vi "Main.vi"() -> ()   [LabVIEW 2024, in "Application.lvlib"]
doc: "This VI is the main application VI in the DQMH project template. This application VI is implemented as a simple state machine, which communicates with two different DQMH modules.\n_____\nBased on DQMH Dev Tools: Project Template 7.1.0.1503."
uses:
  Application.lvlib
  Application Data--cluster.ctl
  State--enum.ctl
  <vilib>/Utility/error.llb/DialogType.ctl
  Camera/Camera.lvlib
  GUI/GUI.lvlib
panel:
  in  "About DQMH":bool
  out "version":string
  in  "Hide GUI Module":bool
  in  "Show GUI Module":bool
  in  "Hide Camera Module":bool
  in  "Show Camera Module":bool
  in  "Stop Camera Module":bool
  in  "Stop GUI Module":bool
  in  "Start GUI Module":bool
  out "Active Camera Modules":string[](array[string])
  in  "Start New Instance Camera Module":bool
  in  "Select Camera Module Instance":i32(ring)=-1 items=["All"=-1, "1"=1]
  out "GUI Running?":bool
  out "Status":string
  # "This top-level application allows you to launch and control a singleton module, and multiple instances of a cloneable module."
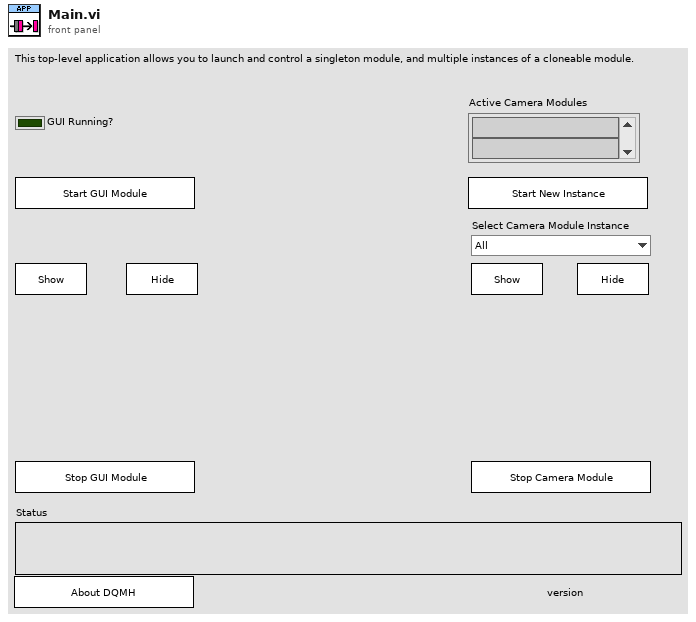
[diagram p1: front panel]
types:
  T1 = typedef "Application.lvlib/State--enum.ctl" = enum16{"Initialize", "Initialize Panel", "UI Interlocks", "Update Status", "Wait for Event", "Exit"}
  T2 = typedef "Application.lvlib/Application Data--cluster.ctl" = cluster{"Status":string, "Singleton Controls":refnum<vi>[], "Cloneable Controls":refnum<vi>[], "Module Ring Value":i32}
  T3 = typedef "Camera.lvlib/Broadcast Events--cluster.ctl" = cluster{"Module Did Init":refnum<user-event>, "Status Updated":refnum<user-event>, "Error Reported":refnum<user-event>, "Module Did Stop":refnum<user-event>, "Update Module Execution Status":refnum<user-event>}
  T4 = typedef "GUI.lvlib/Broadcast Events--cluster.ctl" = cluster{"Module Did Init":refnum<user-event>, "Status Updated":refnum<user-event>, "Error Reported":refnum<user-event>, "Module Did Stop":refnum<user-event>, "Update Module Execution Status":refnum<user-event>, "Update References":refnum<user-event>}
  T5 = enum8{"Enabled", "Disabled", "Disabled and Grayed Out"}
  T6 = typedef "DialogType.ctl" = u16
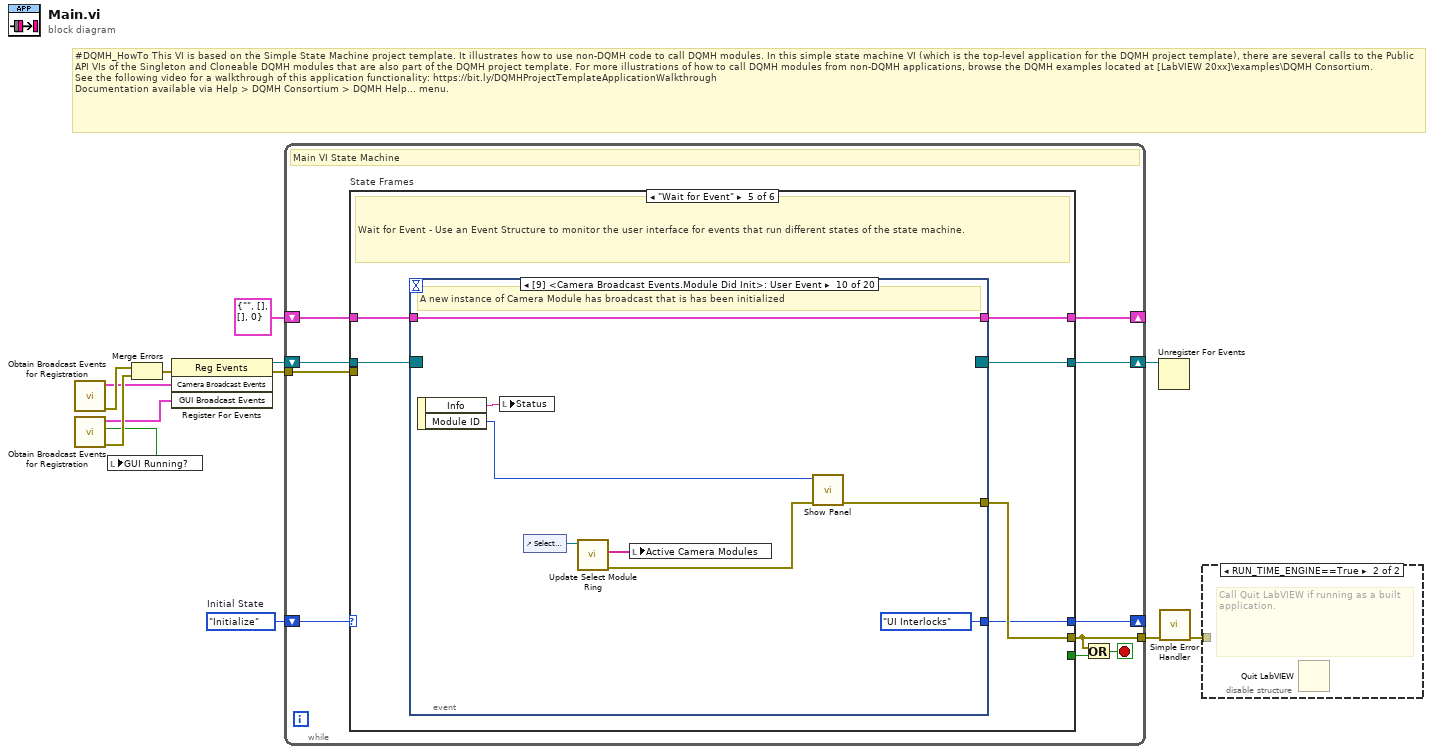
[diagram p0: block diagram]
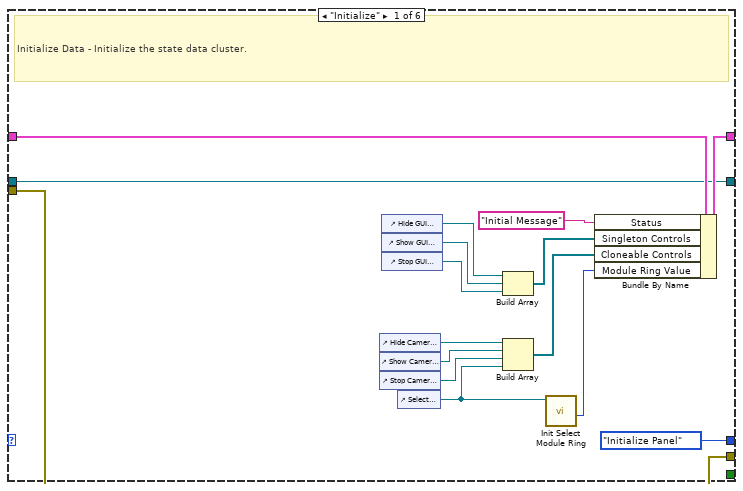
[diagram p2: hidden frame]
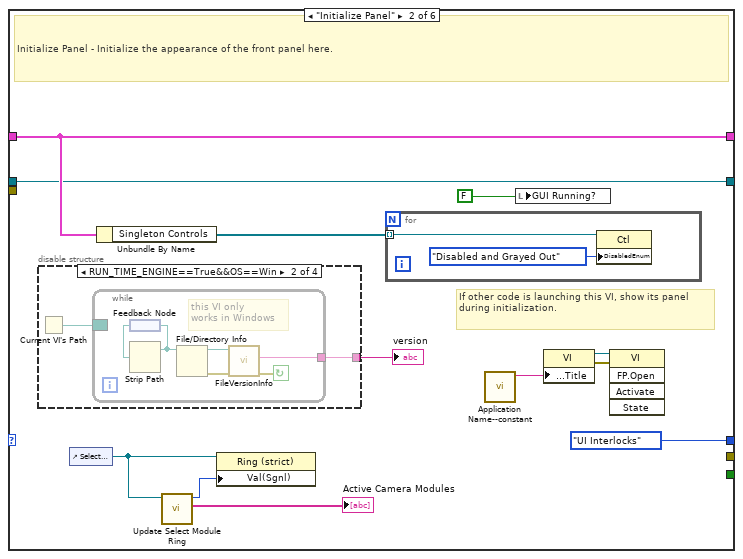
[diagram p3: hidden frame]
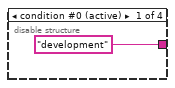
[diagram p4: hidden frame]
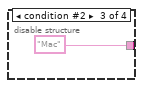
[diagram p5: hidden frame]
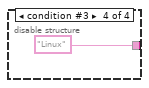
[diagram p6: hidden frame]
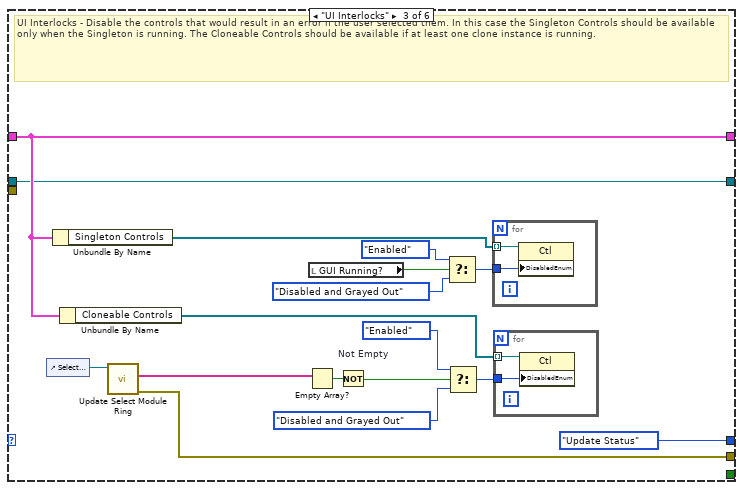
[diagram p7: hidden frame]
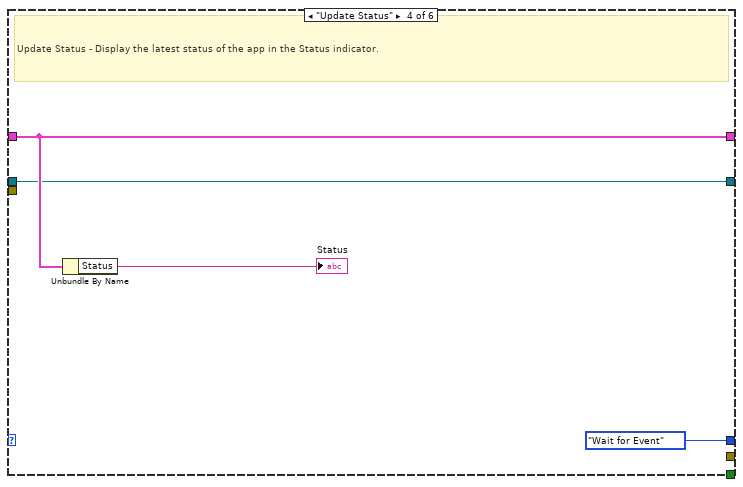
[diagram p8: hidden frame]
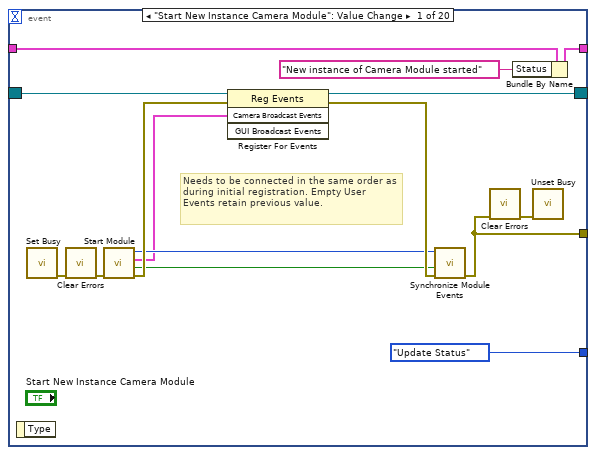
[diagram p9: hidden frame]
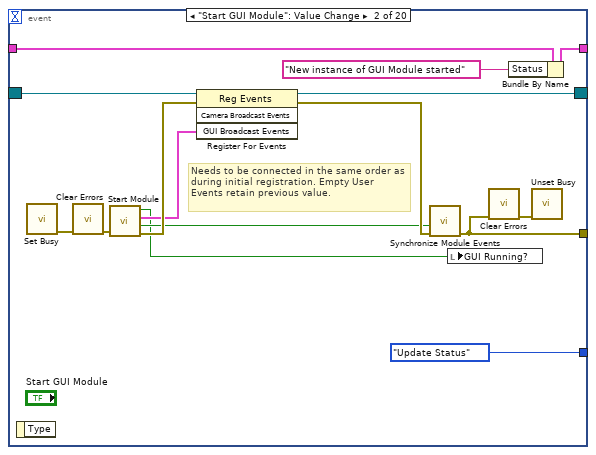
[diagram p10: hidden frame]
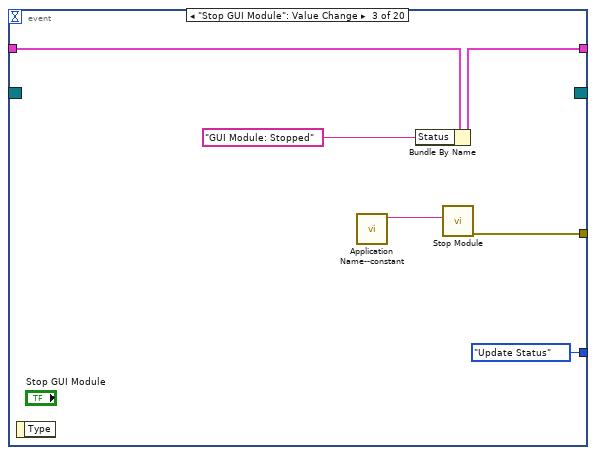
[diagram p11: hidden frame]
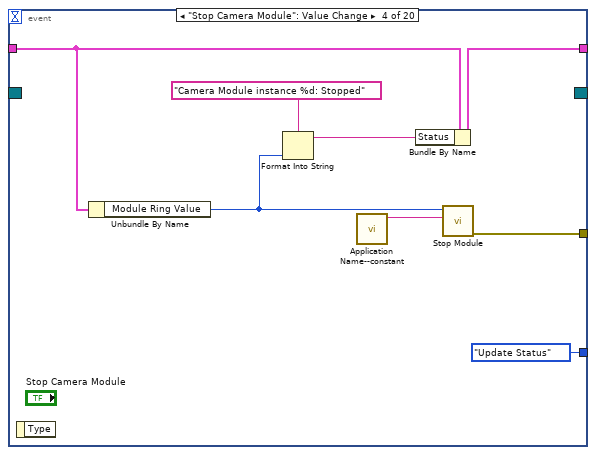
[diagram p12: hidden frame]
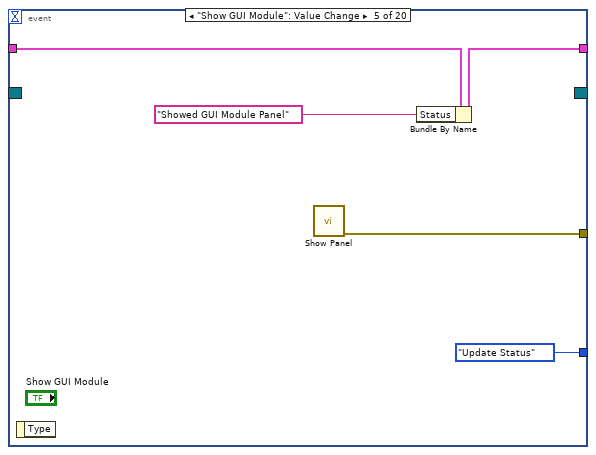
[diagram p13: hidden frame]
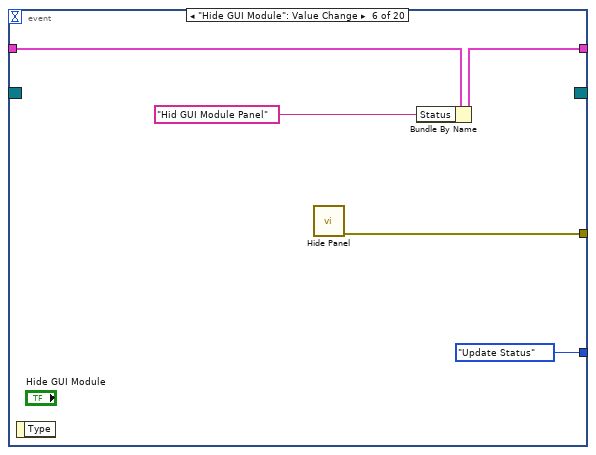
[diagram p14: hidden frame]
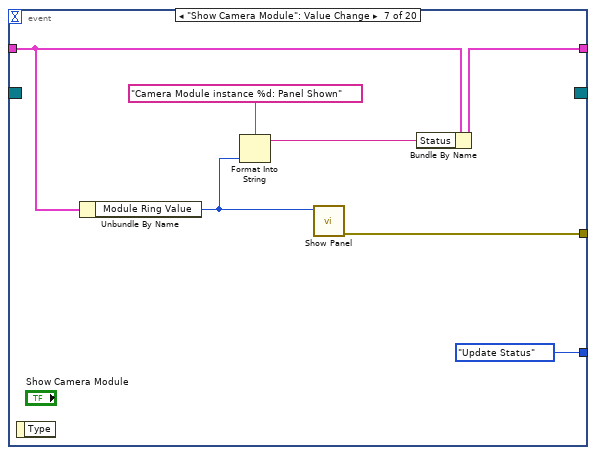
[diagram p15: hidden frame]
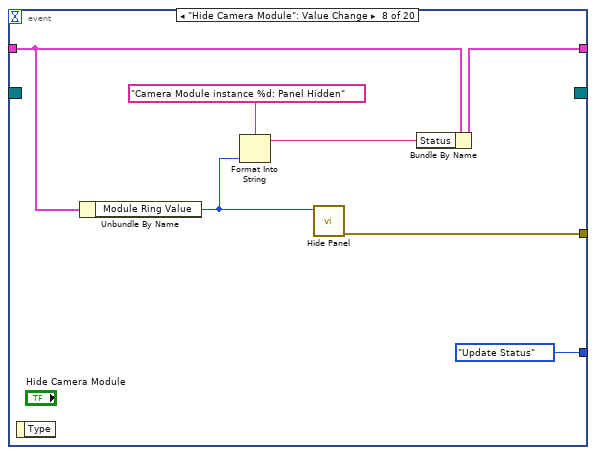
[diagram p16: hidden frame]
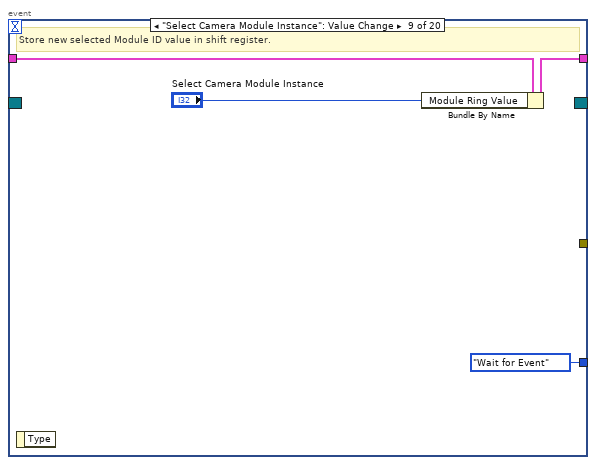
[diagram p17: hidden frame]
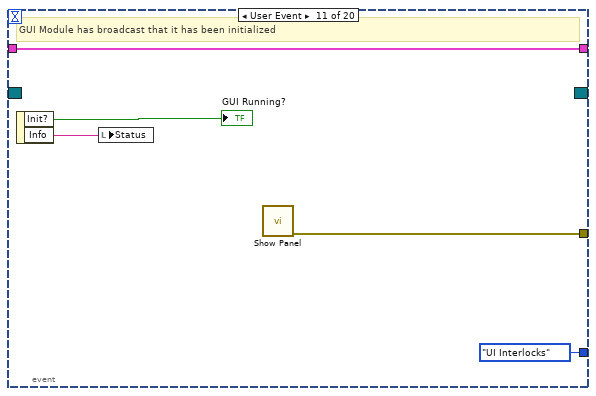
[diagram p18: hidden frame]
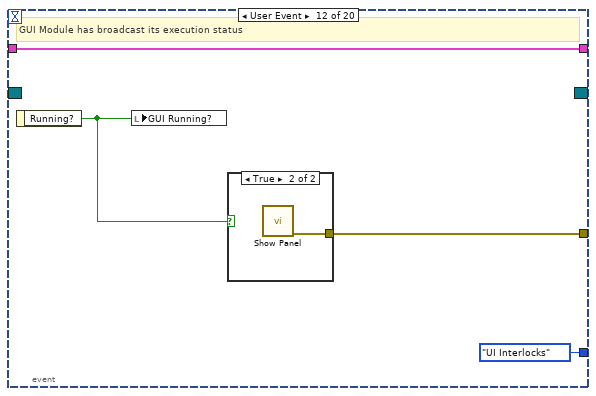
[diagram p19: hidden frame]
diagram:
  w4 = State--enum."Initialize"  # Initial State
  # "#DQMH_HowTo This VI is based on the Simple State Machine project template. It illustrates how to use non-DQMH code to call DQMH modules. In this simple state machine VI (which is the top-level application for the DQMH project template), there are several calls to the Public API VIs of the Singleton and Cloneable DQMH modules that are also part of the DQMH project template. For more illustrations of how to call DQMH modules from non-DQMH applications, browse the DQMH examples located at [LabVIEW 20xx]\\examples\\DQMH Consortium.\nSee the following video for a walkthrough of this application functionality: https://bit.ly/DQMHProjectTemplateApplicationWalkthrough\nDocumentation available via Help > DQMH Consortium > DQMH Help... menu."
  n1 = call "Obtain Broadcast Events for Registration.vi"() -> ("error out"=w9:errorcluster, "Camera Broadcast Events"=w6:T3)  [unwired: 9 in, 1 out]
  n2 = call "Obtain Broadcast Events for Registration.vi"() -> ("error out"=w8:errorcluster, "Already running?"=w1:bool, "GUI Broadcast Events"=w5:T4)  [unwired: 9 in]
  n3 = local write "GUI Running?"(w1) -> ()
  n4 = Merge Errors(w9, w8) -> (w10:errorcluster)
  n5 = register-events(error in=w10, w6, w5) -> (reference out=w3:refnum<event-registration>, error out=w11:errorcluster)  [unwired: 1 in]
  n6 = while {
    shift-right: [w20] -> _
    shift-left: T2 {"Status"="", "Singleton Controls"=[], "Cloneable Controls"=[], "Module Ring Value"=0} ("Data Cluster") -> [w21]
    tunnel: [w23] -> w13
    shift-right: [w16] -> _
    shift-left: w4 -> [w18]
    shift-right: [w14] -> w2
    shift-left: w3 -> [w15]
    tunnel: w11 -> [w22]
    stop <- w17 stop-if-true
    # "Main VI State Machine"
    n7 = case "State Frames" shown="\"Wait for Event\"" w18 {
      tunnel: [w39 _ w81 _ w95 w249] -> w23
      tunnel: w21 -> [w38 w48 w69 w89 w92 w246]
      tunnel: [w37 w48 w69 w89 w91 w246] -> w20
      tunnel: [_ _ _ _ _ w245] -> w19
      tunnel: [State--enum."Initialize Panel" ("State") State--enum."UI Interlocks" ("State") State--enum."Update Status" ("State") State--enum."Wait for Event" ("State") w90 State--enum."Exit" ("State")] -> w16
      tunnel: w15 -> [w24 w45 w65 w86 w94 w243]
      tunnel: [w24 w45 w65 w86 w93 w243] -> w14
      tunnel: w22 -> [w39 _ _ _ _ _]
      frame "Initialize" {
        # "Initialize Data - Initialize the state data cluster."
        n8 = control-ref of="Hide Camera Module"() -> (w31:refnum<vi>)
        n9 = control-ref of="Show Camera Module"() -> (w30:refnum<vi>)
        n10 = control-ref of="Stop Camera Module"() -> (w29:refnum<vi>)
        n11 = control-ref of="Hide GUI Module"() -> (w35:refnum<vi>)
        n12 = control-ref of="Show GUI Module"() -> (w34:refnum<vi>)
        n13 = control-ref of="Stop GUI Module"() -> (w33:refnum<vi>)
        n14 = control-ref of="Select Camera Module Instance"() -> (w26:refnum<vi>)
        n15 = Build Array(w35, w34, w33) -> (w32:refnum<vi>[])
        n16 = Build Array(w31, w30, w29, w26) -> (w28:refnum<vi>[])
        n17 = call "Init Select Module Ring.vi"("Select Module Ring Ref"=w26) -> ("Module Ring Value"=w25:i32)  [unwired: 8 in, 2 out]
        n18 = Bundle By Name(cluster=w38, "Status"="Initial Message" ("Initial Message"), "Singleton Controls"=w32, "Cloneable Controls"=w28, "Module Ring Value"=w25) -> (w37:T2)
      }
      frame "Initialize Panel" {
        # "If other code is launching this VI, show its panel during initialization."
        # "Initialize Panel - Initialize the appearance of the front panel here."
        n19 = disable-structure "Conditional Disable Structure" shown="RUN_TIME_ENGINE==True&&OS==Win" {
          disable-tunnel: ["development" w53 "Mac" "Linux"] -> w42
          frame condition #0 (active) {
          }
          frame condition #1 {
            n20 = Current VI's Path() -> (path=w54:path)
            n21 = while {
              border: w54 -> [_]
              tunnel: [w55] -> w53
              stop <- w59 continue-if-true
              # "this VI only \nworks in Windows"
              n22 = feedback #1() -> (w58:path)
              n23 = Strip Path(path=w58) -> (stripped path=w57:path)  [unwired: 1 out]
              n24 = feedback-in #1(w57) -> ()
              n25 = File/Directory Info(path=w57) -> (path out=w56:path, error out=w60:errorcluster)  [unwired: 1 in, 5 out]
              n26 = call <vilib>:"FileVersionInfo.vi"("error in (no error)"=w60, "Application Path in"=w56) -> ("error out"=w59:errorcluster, "File Version Info"=w55:string)  [unwired: 6 in, 2 out]
            }
          }
          frame condition #2 {
          }
          frame condition #3 {
          }
        }
        "version" <- w42
        n27 = control-ref of="Select Camera Module Instance"() -> (w44:refnum<vi>)
        n28 = Unbundle By Name(w48) -> ("Singleton Controls"=w47:refnum<vi>[])
        n29 = call "Update Select Module Ring.vi"("Select Module Ring Ref"=w44) -> ("Active Modules (Array)"=→"Active Camera Modules":string[], "New Module Ring Value"=w43:i32)  [unwired: 8 in, 1 out]
        n30 = property on="Property Node" class="Ring (strict)"(reference=w44, "Val(Sgnl)"=w43) -> ()  [unwired: 1 in, 2 out]
        n31 = for {
          tunnel: w47 -> [w64] mode=indexing
          n32 = property on="Property Node" class="Ctl"(reference=w64, "DisabledEnum"=T5."Disabled and Grayed Out" ("Disabled")) -> ()  [unwired: 1 in, 2 out]
        }
        n33 = call "Application Name--constant.vi"() -> ("Application Name"=w41:string)  [unwired: 11 in]
        n34 = local write "GUI Running?"(FALSE ("My Singleton Module Init?")) -> ()
        n35 = property on="Property Node" class="VI"("Front Panel.Title"=w41) -> (reference out=w40:refnum<vi>, error out=w51:errorcluster)  [unwired: 2 in]
        n36 = invoke class="VI" method="FP.Open"(reference=w40, error in=w51) -> ()  [unwired: 3 in, 5 out]
      }
      frame "UI Interlocks" {
        # "UI Interlocks - Disable the controls that would result in an error if the user selected them. In this case the Singleton Controls should be available only when the Singleton is running. The Cloneable Controls should be available if at least one clone instance is running."
        n37 = control-ref of="Select Camera Module Instance"() -> (w80:refnum<vi>)
        n38 = Unbundle By Name(w69) -> ("Singleton Controls"=w74:refnum<vi>[])
        n39 = Unbundle By Name(w69) -> ("Cloneable Controls"=w68:refnum<vi>[])
        n40 = call "Update Select Module Ring.vi"("Select Module Ring Ref"=w80) -> ("error out"=w81:errorcluster, "Active Modules (Array)"=w79:string[])  [unwired: 8 in, 1 out]
        n41 = Empty Array?(array=w79) -> (empty?=w78:bool)
        n42 = local read "GUI Running?"() -> (w73:bool)
        n43 = Not "Not Empty"(x=w78) -> (.not. x?=w67:bool)
        n44 = Select(t=T5."Enabled" ("Disabled"), s=w73, f=T5."Disabled and Grayed Out" ("Disabled")) -> (s? t:f=w75:T5)
        n45 = Select(t=T5."Enabled" ("Disabled"), s=w67, f=T5."Disabled and Grayed Out" ("Disabled")) -> (s? t:f=w72:T5)
        n46 = for {
          tunnel: w74 -> [w85] mode=indexing
          tunnel: w75 -> [w84]
          n47 = property on="Property Node" class="Ctl"(reference=w85, "DisabledEnum"=w84) -> ()  [unwired: 1 in, 2 out]
        }
        n48 = for {
          tunnel: w68 -> [w83] mode=indexing
          tunnel: w72 -> [w82]
          n49 = property on="Property Node" class="Ctl"(reference=w83, "DisabledEnum"=w82) -> ()  [unwired: 1 in, 2 out]
        }
      }
      frame "Update Status" {
        # "Update Status - Display the latest status of the app in the Status indicator."
        n50 = Unbundle By Name(w89) -> ("Status"=→"Status":string)
      }
      frame "Wait for Event" {
        # "Wait for Event - Use an Event Structure to monitor the user interface for events that run different states of the state machine."
        n51 = event shown="[9] <Camera Broadcast Events.Module Did Init>: User Event" {
          selector: w94 -> [w102 w118 _ _ _ _ _ _ _ _ _ _ _ _ _ _ _ _ _ _]
          dyn-events: [w101 w117 _ _ _ _ _ _ _ _ _ _ _ _ _ _ _ _ _ _] -> w93
          timeout: _ -> [_ _ _ _ _ _ _ _ _ _ _ _ _ _ _ _ _ _ _ _]
          tunnel: [w110 w125 w131 w139 w144 w149 w156 w163 _ w175 w180 w184 _ _ _ _ w226 _ _ w237] -> w95
          tunnel: [w97 w114 w127 w136 w142 w147 w155 w162 w165 w169 w177 w183 w186 w191 w206 w215 w219 w230 w235 w239] -> w91
          tunnel: w92 -> [w98 w115 w128 w135 w143 w148 w153 w160 w166 w169 w177 w183 w187 w192 w207 w216 w222 w231 w235 w239]
          tunnel: [State--enum."Update Status" ("State") State--enum."Update Status" ("State") State--enum."Update Status" ("State") State--enum."Update Status" ("State") State--enum."Update Status" ("State") State--enum."Update Status" ("State") State--enum."Update Status" ("State") State--enum."Update Status" ("State") State--enum."Wait for Event" ("State") State--enum."UI Interlocks" ("State") State--enum."UI Interlocks" ("State") State--enum."UI Interlocks" ("State") State--enum."Update Status" ("State") State--enum."Update Status" ("State") State--enum."Update Status" ("State") State--enum."Update Status" ("State") State--enum."UI Interlocks" ("State") State--enum."UI Interlocks" ("State") State--enum."Exit" ("State") State--enum."Wait for Event" ("State")] -> w90
          event "Start New Instance Camera Module": Value Change {
            # "Needs to be connected in the same order as during initial registration. Empty User Events retain previous value."
            n52 = event-data() -> ()  [unwired: 1 in, 1 out]
            n53 = call <vilib>:"Set Busy.vi"() -> ("error out"=w106:errorcluster)  [unwired: 10 in, 1 out]
            n54 = call <vilib>:"Clear Errors.vi"("error in (no error)"=w106) -> ("error out"=w107:errorcluster)  [unwired: 5 in, 1 out]
            n55 = call "Start Module.vi"("error in"=w107) -> ("error out"=w109:errorcluster, "Wait for Event Sync?"=w104:bool, "Camera Broadcast Events"=w100:T3, "Module ID"=w103:i32)  [unwired: 6 in, 1 out]
            n56 = register-events(reference=w102, error in=w109, w100) -> (reference out=w101:refnum<event-registration>, error out=w108:errorcluster)  [unwired: 1 in]
            n57 = call "Synchronize Module Events.vi"("error in"=w108, "Wait for Event Sync?"=w104, "Module ID in"=w103) -> ("error out"=w110:errorcluster)  [unwired: 7 in, 1 out]
            n58 = call <vilib>:"Clear Errors.vi"("error in (no error)"=w110) -> ("error out"=w105:errorcluster)  [unwired: 5 in, 1 out]
            n59 = Bundle By Name(cluster=w98, "Status"="New instance of Camera Module started") -> (w97:T2)
            n60 = call <vilib>:"Unset Busy.vi"("error in (no error)"=w105) -> ()  [unwired: 10 in, 1 out]
          }
          event "Start GUI Module": Value Change {
            # "Needs to be connected in the same order as during initial registration. Empty User Events retain previous value."
            n61 = event-data() -> ()  [unwired: 1 in, 1 out]
            n62 = call <vilib>:"Set Busy.vi"() -> ("error out"=w121:errorcluster)  [unwired: 10 in, 1 out]
            n63 = call <vilib>:"Clear Errors.vi"("error in (no error)"=w121) -> ("error out"=w122:errorcluster)  [unwired: 5 in, 1 out]
            n64 = call "Start Module.vi"("error in"=w122) -> ("error out"=w124:errorcluster, "Wait for Event Sync?"=w119:bool, "GUI Broadcast Events"=w112:T4, "Module Was Already Running?"=w111:bool)  [unwired: 6 in, 1 out]
            n65 = register-events(reference=w118, error in=w124, w112) -> (reference out=w117:refnum<event-registration>, error out=w123:errorcluster)  [unwired: 1 in]
            n66 = call "Synchronize Module Events.vi"("error in"=w123, "Wait for Event Sync?"=w119) -> ("error out"=w125:errorcluster)  [unwired: 9 in]
            n67 = local write "GUI Running?"(w111) -> ()
            n68 = call <vilib>:"Clear Errors.vi"("error in (no error)"=w125) -> ("error out"=w120:errorcluster)  [unwired: 5 in, 1 out]
            n69 = Bundle By Name(cluster=w115, "Status"="New instance of GUI Module started") -> (w114:T2)
            n70 = call <vilib>:"Unset Busy.vi"("error in (no error)"=w120) -> ()  [unwired: 10 in, 1 out]
          }
          event "Stop GUI Module": Value Change {
            n71 = event-data() -> ()  [unwired: 1 in, 1 out]
            n72 = call "Application Name--constant.vi"() -> ("Application Name"=w129:string)  [unwired: 11 in]
            n73 = Bundle By Name(cluster=w128, "Status"="GUI Module: Stopped" ("Message")) -> (w127:T2)
            n74 = call "Stop Module.vi"("Origin"=w129) -> ("error out"=w131:errorcluster)  [unwired: 10 in]
          }
          event "Stop Camera Module": Value Change {
            n75 = event-data() -> ()  [unwired: 1 in, 1 out]
            n76 = Unbundle By Name(w135) -> ("Module Ring Value"=w132:i32)
            n77 = Format Into String(format string="Camera Module instance %d: Stopped" ("Message"), w132) -> (resulting string=w133:string)  [unwired: 2 in, 1 out]
            n78 = call "Application Name--constant.vi"() -> ("Application Name"=w137:string)  [unwired: 11 in]
            n79 = Bundle By Name(cluster=w135, "Status"=w133) -> (w136:T2)
            n80 = call "Stop Module.vi"("Origin"=w137, "Module ID"=w132) -> ("error out"=w139:errorcluster)  [unwired: 9 in]
          }
          event "Show GUI Module": Value Change {
            n81 = event-data() -> ()  [unwired: 1 in, 1 out]
            n82 = call "Show Panel.vi"() -> ("error out"=w144:errorcluster)  [unwired: 11 in]
            n83 = Bundle By Name(cluster=w143, "Status"="Showed GUI Module Panel" ("Message")) -> (w142:T2)
          }
          event "Hide GUI Module": Value Change {
            n84 = event-data() -> ()  [unwired: 1 in, 1 out]
            n85 = call "Hide Panel.vi"() -> ("error out"=w149:errorcluster)  [unwired: 11 in]
            n86 = Bundle By Name(cluster=w148, "Status"="Hid GUI Module Panel" ("Message")) -> (w147:T2)
          }
          event "Show Camera Module": Value Change {
            n87 = event-data() -> ()  [unwired: 1 in, 1 out]
            n88 = Unbundle By Name(w153) -> ("Module Ring Value"=w151:i32)
            n89 = Format Into String(format string="Camera Module instance %d: Panel Shown" ("Message"), w151) -> (resulting string=w150:string)  [unwired: 2 in, 1 out]
            n90 = call "Show Panel.vi"("Module ID"=w151) -> ("error out"=w156:errorcluster)  [unwired: 10 in]
            n91 = Bundle By Name(cluster=w153, "Status"=w150) -> (w155:T2)
          }
          event "Hide Camera Module": Value Change {
            n92 = event-data() -> ()  [unwired: 1 in, 1 out]
            n93 = Unbundle By Name(w160) -> ("Module Ring Value"=w158:i32)
            n94 = Format Into String(format string="Camera Module instance %d: Panel Hidden" ("Message"), w158) -> (resulting string=w157:string)  [unwired: 2 in, 1 out]
            n95 = call "Hide Panel.vi"("Module ID"=w158) -> ("error out"=w163:errorcluster)  [unwired: 10 in]
            n96 = Bundle By Name(cluster=w160, "Status"=w157) -> (w162:T2)
          }
          event "Select Camera Module Instance": Value Change {
            # "Store new selected Module ID value in shift register."
            n97 = event-data() -> ()  [unwired: 1 in, 1 out]
            n98 = Bundle By Name(cluster=w166, "Module Ring Value"="Select Camera Module Instance") -> (w165:T2)
          }
          event User Event {
            # "A new instance of Camera Module has broadcast that is has been initialized"
            n99 = event-data() -> ("Info"=w173:string, "Module ID"=w168:i32)  [unwired: 1 in]
            n100 = local write "Status"(w173) -> ()
            n101 = control-ref of="Select Camera Module Instance"() -> (w172:refnum<vi>)
            n102 = call "Update Select Module Ring.vi"("Select Module Ring Ref"=w172) -> ("error out"=w174:errorcluster, "Active Modules (Array)"=w171:string[])  [unwired: 8 in, 1 out]
            n103 = local write "Active Camera Modules"(w171) -> ()
            n104 = call "Show Panel.vi"("error in"=w174, "Module ID"=w168) -> ("error out"=w175:errorcluster)  [unwired: 9 in]
          }
          event User Event {
            # "GUI Module has broadcast that it has been initialized"
            n105 = event-data() -> ("Init?"=→"GUI Running?":bool, "Info"=w179:string)  [unwired: 1 in]
            n106 = local write "Status"(w179) -> ()
            n107 = call "Show Panel.vi"() -> ("error out"=w180:errorcluster)  [unwired: 11 in]
          }
          event User Event {
            # "GUI Module has broadcast its execution status"
            n108 = event-data() -> ("Running?"=w181:bool)  [unwired: 1 in]
            n109 = local write "GUI Running?"(w181) -> ()
            n110 = case shown="True" w181 {
              tunnel: [_ w185] -> w184
              frame False {
              }
              frame True {
                n111 = call "Show Panel.vi"() -> ("error out"=w185:errorcluster)  [unwired: 11 in]
              }
            }
          }
          event User Event {
            # "An instance of Camera Module has broadcast its status"
            n112 = event-data() -> ("Status"=w189:string)  [unwired: 1 in]
            n113 = Bundle By Name(cluster=w187, "Status"=w189) -> (w186:T2)
          }
          event User Event {
            # "GUI Module has broadcast its status"
            n114 = event-data() -> ("Status"=w193:string)  [unwired: 1 in]
            n115 = Bundle By Name(cluster=w192, "Status"=w193) -> (w191:T2)
          }
          event User Event {
            w198 = T6 0 items=["no dialog", "OK message", "continue or stop message", "OK message + warnings", "continue/stop + warnings"] ("type of dialog (OK msg:1)")
            # "Camera Module had an error"
            n116 = event-data() -> ("Module Name"=w195:string, "Additional Information"=w196:string, "Error"=w197:errorcluster)  [unwired: 1 in]
            n117 = call <vilib>:"Space Constant.vi"() -> ("String"=w202:string)
            n118 = call <vilib>:"Simple Error Handler.vi"("type of dialog (OK msg:1)"=w198, "error in (no error)"=w197) -> ("message"=w199:string)  [unwired: 3 in, 4 out]
            n119 = call <vilib>:"Search and Replace Pattern.vi"("string"=w199, "regular expression (\"\")"="[\\r\\n]" ("regular expression (\"\")"), "replace string (\"\")"=w202, "replace all? (F)"=TRUE ("replace all CR/LF with spaces")) -> ("result string"=w200:string)  [unwired: 1 in, 1 out]
            n120 = Format Into String(format string="%s: %s Additional Information: %s", w195, w200, w196) -> (resulting string=w194:string)  [unwired: 2 in, 1 out]
            n121 = Bundle By Name(cluster=w207, "Status"=w194) -> (w206:T2)
          }
          event User Event {
            # "GUI Module had an error"
            n122 = event-data() -> ("Module Name"=w209:string, "Additional Information"=w213:string, "Error"=w217:errorcluster)  [unwired: 1 in]
            n123 = Unbundle By Name(w217) -> ("code"=w208:i32, "source"=w212:string)
            n124 = Format Into String(format string="Error code %d Module: %s  Additional Information: %s\nSource: %s", w208, w209, w213, w212) -> (resulting string=w210:string)  [unwired: 2 in, 1 out]
            n125 = Bundle By Name(cluster=w216, "Status"=w210) -> (w215:T2)
          }
          event User Event {
            n126 = event-data() -> ("Origin"=w221:string)  [unwired: 1 in]
            n127 = Bundle By Name(cluster=w222, "Status"=w221) -> (w220:T2)
            n128 = control-ref of="Select Camera Module Instance"() -> (w225:refnum<vi>)
            n129 = call "Update Select Module Ring.vi"("Select Module Ring Ref"=w225) -> ("error out"=w226:errorcluster, "Active Modules (Array)"=w224:string[], "New Module Ring Value"=w218:i32)  [unwired: 8 in]
            n130 = Bundle By Name(cluster=w220, "Module Ring Value"=w218) -> (w219:T2)
            n131 = local write "Active Camera Modules"(w224) -> ()
          }
          event User Event {
            n132 = event-data() -> ("Origin"=w228:string)  [unwired: 1 in]
            n133 = local write "GUI Running?"(FALSE ("My Singleton Module Init?")) -> ()
            n134 = Concatenate Strings(w228, " Did Stop.") -> (w227:string)
            n135 = Bundle By Name(cluster=w231, "Status"=w227) -> (w230:T2)
          }
          event Panel Close? {
            # "Go to the 'Exit' state if the user tries to close the panel."
            n136 = event-data() -> ()  [unwired: 1 in, 1 out]
            n137 = event-data ("Event Filter Node")("Discard?"=TRUE) -> ()  [unwired: 1 in, 1 out]
          }
          event "About DQMH": Value Change {
            # "Display DQMH About Box"
            n138 = event-data() -> ()  [unwired: 1 in, 1 out]
            n139 = call <vilib>:"DQMH_About Box.vi"() -> ("error out"=w237:errorcluster)  [unwired: 11 in]
          }
        }
      }
      frame "Exit" {
        w240 = TRUE  # Wait for Module to stop?
        w245 = TRUE  # Stop the VI
        # "Stop all modules launched"
        # "Exit - Exit the application."
        n140 = call "Application Name--constant.vi"() -> ("Application Name"=w241:string)  [unwired: 11 in]
        n141 = call "Stop Module.vi"("Wait for Module to stop? (F)"=w240, "Origin"=w241, "Module ID"=-1) -> ("error out"=w247:errorcluster)  [unwired: 8 in]
        n142 = call "Stop Module.vi"("Wait for Module to Stop? (F)"=w240, "Origin"=w241) -> ("error out"=w248:errorcluster)  [unwired: 9 in]
        n143 = Merge Errors(w247, w248) -> (w249:errorcluster)
      }
    }
    n144 = Or(x=w23, y=w19) -> (x .or. y?=w17:bool)
  }
  n145 = Unregister For Events(event registration refnum=w2) -> ()  [unwired: 1 in, 1 out]
  n146 = call <vilib>:"Simple Error Handler.vi"("error in (no error)"=w13) -> ("error out"=w12:errorcluster)  [unwired: 4 in, 4 out]
  n147 = disable-structure "Conditional Disable Structure" shown="RUN_TIME_ENGINE==True" {
    disable-tunnel: w12 -> [_ _]
    frame condition #0 (active) {
    }
    frame condition #1 {
      # "Call Quit LabVIEW if running as a built application."
      n148 = Quit LabVIEW() -> ()  [unwired: 1 in]
    }
  }
